vi "Read CSM Module Info.vi"(6 "Config Path":path, 8 "error in (no error)":errorcluster, 11 "CSM Name":string) -> (0 "error out":errorcluster, 3 "Cluster":cluster{"VIName":string})   [LabVIEW 2017, in "CSM-Helper API with lvcsm Support.lvlib"]
uses:
  CSM-Helper API with lvcsm Support.lvlib
  <vilib>/Utility/config.llb/Read Key (String).vi
  <vilib>/Utility/config.llb/NI_LVConfig.lvlib
  lvcsmFile/lvcsm File Support.lvlib
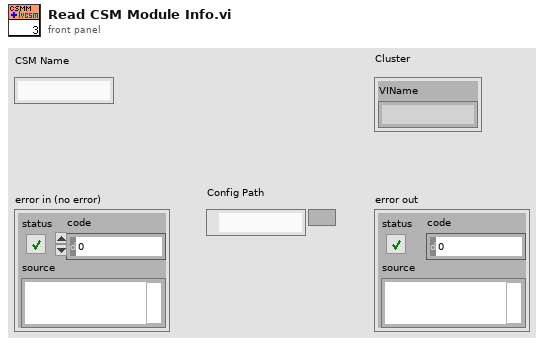
[diagram p1: front panel]
types:
  T1 = typedef "NI_LVConfig.lvlib/Config Data RefNum.ctl" = refnum<k1>
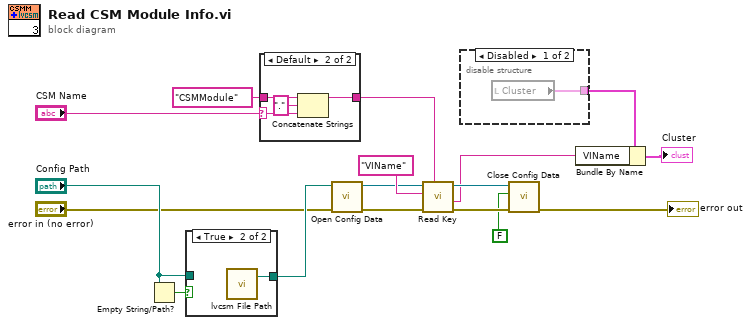
[diagram p0: block diagram]
diagram:
  n1 = Empty String/Path?(string/path="Config Path") -> (empty?=w15:bool)
  n2 = case shown="True" w15 {
    tunnel: [w18 w19] -> w17
    tunnel: "Config Path" -> [w18 _]
    frame False {
    }
    frame True {
      n3 = call "lvcsm File Path.vi"() -> ("Appended Path"=w19:path)  [unwired: 3 in]
    }
  }
  n4 = case shown="Default" "CSM Name" {
    selector: "CSM Name" -> [_ w22]
    tunnel: "CSMModule" ("Section Prefix") -> [w20 w24]
    tunnel: [w20 w23] -> w9
    frame "" {
    }
    frame Default {
      n5 = Concatenate Strings(w24, "." ("string"), w22) -> (w23:string)
    }
  }
  n6 = call <vilib>:"Open Config Data.vi"("error in (no error)"="error in (no error)", "configuration file path"=w17) -> ("error out"=w5:errorcluster, "refnum"=w6:T1)  [unwired: 7 in, 1 out]
  n7 = call-poly <vilib>:"Read Key.vi"("section"=w9, "error in (no error)"=w5, "key"="VIName", "refnum"=w6) -> ("error out"=w7:errorcluster, "value"=w2:string, "refnum out"=w8:T1)  [unwired: 4 in, 1 out]
  n8 = disable-structure shown="Disabled" {
    disable-tunnel: [w25 _] -> w3
    frame Disabled {
      n9 = local read "Cluster"() -> (w25:cluster{"VIName":string})
    }
    frame Enabled {
    }
  }
  n10 = call <vilib>:"Close Config Data.vi"("error in (no error)"=w7, "write file if changed (T)"=FALSE, "refnum"=w8) -> ("error out"=→"error out":errorcluster)  [unwired: 7 in, 1 out]
  n11 = Bundle By Name(cluster=w3, "VIName"=w2) -> (→"Cluster":cluster{"VIName":string})
